vi "initialize-data.vi"(8 "error in (no error)":errorcluster, 9 "store_method":T1=enum."fixed", 10 "y_axis":dbl[][](array[numeric]), 11 "x_axis":dbl[](array[numeric])) -> (0 "error out":errorcluster, 3 "dvr":refnum<data-value>)   [LabVIEW 2015, in "lv-graph-global.lvlib"]
doc: "Initialize can be used to configure how much data can be stored and what happens when that max is reached. Use this to configure the expected number of rows, columns and the store method."
uses:
  _controls/data.ctl
  _controls/configuration.ctl
  _controls/store_method.ctl
  lv-graph-global.lvlib
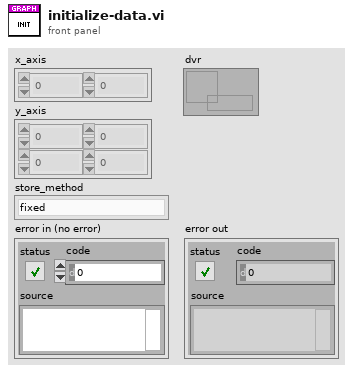
[diagram p1: front panel]
types:
  T1 = typedef "lv-graph-global.lvlib/store_method.ctl" = enum16{"<store_method>", "fixed", "grow"}
  T2 = typedef "lv-graph-global.lvlib/data.ctl" = cluster{"configuration":T3, "index":i32, "x_axis":dbl[], "y_axis":dbl[][]}
  T3 = typedef "lv-graph-global.lvlib/configuration.ctl" = cluster{"store_method":T1, "rows":i32, "columns":i32}
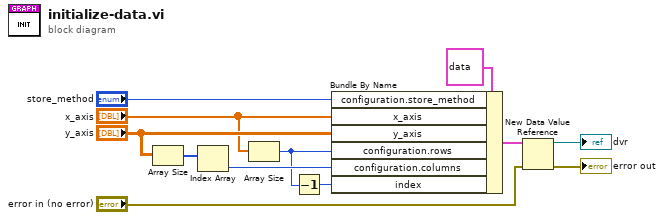
[diagram p0: block diagram]
diagram:
  n1 = Array Size(array="y_axis") -> (size(s)=w4:i32[])
  n2 = Index Array(array=w4) -> (element=w3:i32)  [unwired: 1 in]
  n3 = Array Size(array="x_axis") -> (size(s)=w2:i32)
  n4 = Decrement(x=w2) -> (x-1=w1:i32)
  n5 = Bundle By Name(cluster=T2 {"configuration"={"store_method"=enum."<store_method>", "rows"=-1, "columns"=-1}, "index"=0, "x_axis"=[], "y_axis"=[]} ("data"), "configuration.store_method"="store_method", "x_axis"="x_axis", "y_axis"="y_axis", "configuration.rows"=w2, "configuration.columns"=w3, "index"=w1) -> (w8:T2)
  n6 = New Data Value Reference(data value=w8, error in="error in (no error)") -> (data value reference=→"dvr":refnum<data-value>, error out=→"error out":errorcluster)
